vi "ExSubSnap.vi"(2 "error in (no error)":errorcluster, 3 "Handle Cluster":T1) -> (0 "error out":errorcluster, 1 "Handle Cluster Out":T1)   [LabVIEW 2010]
panel:
  # "ExSubSnapNStore: this VI\nStarts the camera and collects\none image and stores it.\nNote the camera should be in \nAsync mode for this sub vi"
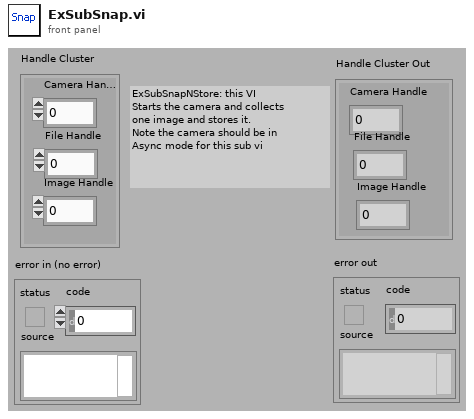
[diagram p1: front panel]
types:
  T1 = cluster{"Camera Handle":u32, "File Handle":u32, "Image Handle":u32}
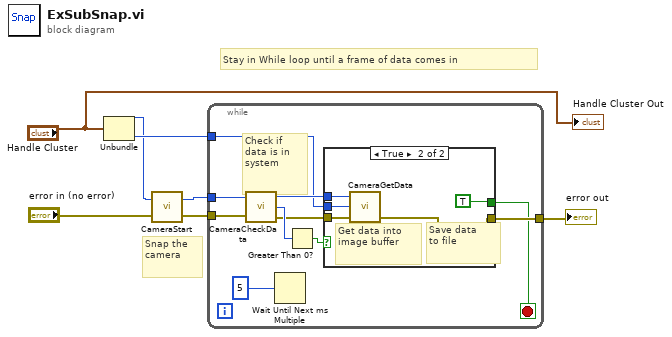
[diagram p0: block diagram]
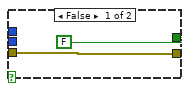
[diagram p2: hidden frame]
diagram:
  # "Snap the\ncamera"
  # "Stay in While loop until a frame of data comes in"
  n1 = Unbundle("Handle Cluster") -> ("Camera Handle"=w5:u32, "Image Handle"=w6:u32)  [unwired: 1 out]
  n2 = call <userlib>:"CameraStart.vi"("error in"="error in (no error)", "Camera Handle"=w5) -> ("error out"=w3:errorcluster, "Camera Handle"=w2:u32)
  n3 = while {
    tunnel: w3 -> [w13]
    tunnel: [w12] -> w7
    tunnel: w6 -> [w11]
    tunnel: w2 -> [w9]
    stop <- w10 stop-if-true
    # "Check if \ndata is in\nsystem"
    n4 = call <userlib>:"CameraCheckData.vi"("Camera Handle"=w9, "error in"=w13) -> ("Camera Handle"=w16:u32, "Number Of Frames Available"=w15:i32, "error out"=w14:errorcluster)
    n5 = Wait Until Next ms Multiple(millisecond multiple=5) -> ()  [unwired: 1 out]
    n6 = Greater Than 0?(x=w15) -> (x > 0?=w17:bool)
    n7 = case shown="True" w17 {
      tunnel: w16 -> [_ w24]
      tunnel: w14 -> [w19 w23]
      tunnel: [w19 w20] -> w12
      tunnel: [FALSE TRUE] -> w10
      tunnel: w11 -> [_ w21]
      frame False {
      }
      frame True {
        # "Save data \nto file"
        # "Get data into\nimage buffer"
        n8 = call <userlib>:"CameraGetData.vi"("error in"=w23, "Data Handle"=w21, "Camera Handle"=w24) -> ("error out"=w20:errorcluster)  [unwired: 2 out]
      }
    }
  }
  "error out" <- w7
  "Handle Cluster Out" <- "Handle Cluster"
